vi "CheckXL_HasThisSheet.vi"(8 "error in (no error)":errorcluster, 10 "SheetName(\"\")":string, 11 "Refnum Cluster In":T1) -> (0 "error out":errorcluster, 2 "Find(False)":bool, 3 "Refnum Out":T1)   [LabVIEW 2015]
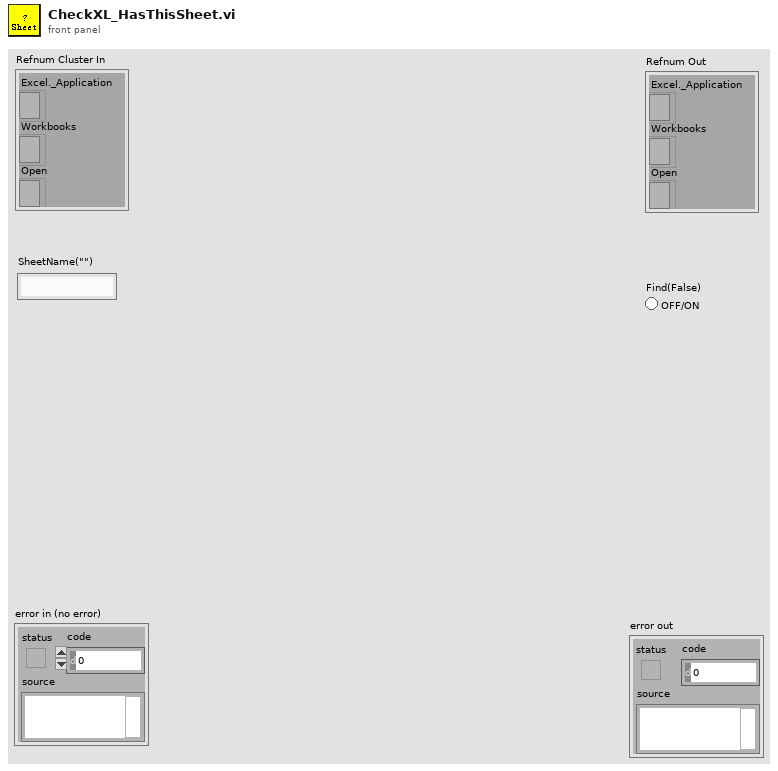
[diagram p1: front panel]
types:
  T1 = cluster{"Excel._Application":refnum<k7>, "Workbooks":refnum<k7>, "Open":refnum<k7>}
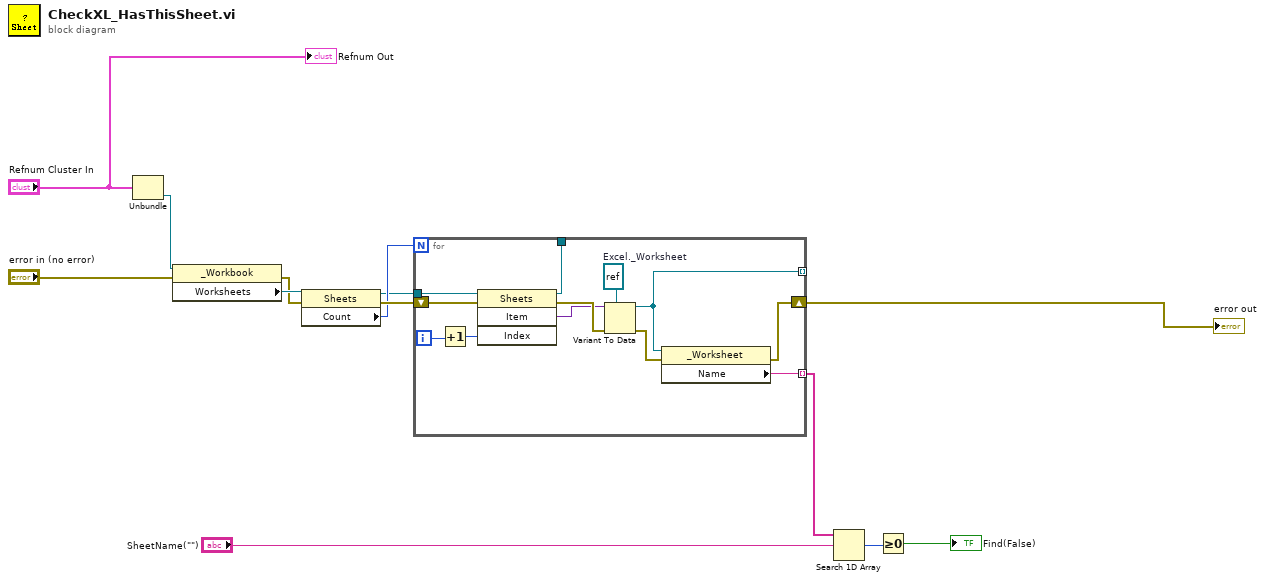
[diagram p0: block diagram]
diagram:
  n1 = Unbundle("Refnum Cluster In") -> ("Open"=w12:refnum<k7>)  [unwired: 2 out]
  n2 = property class="_Workbook"(reference=w12, error in="error in (no error)") -> (error out=w8:errorcluster, "Worksheets"=w9:refnum<k7>)  [unwired: 1 out]
  n3 = property class="Sheets"(reference=w9, error in=w8) -> (reference out=w3:refnum<k7>, error out=w7:errorcluster, "Count"=w6:i32)
  n4 = for {
    N: w6 -> [_]
    tunnel: [w25] -> _
    shift-right: [w19] -> w13
    shift-left: w7 -> [w21]
    tunnel: [w18] -> _ mode=indexing
    tunnel: [w17] -> w5 mode=indexing
    tunnel: w3 -> [w16]
    i -> [w15]
    w23 = refnum<k7> refnum  # Excel._Worksheet
    n5 = Increment(x=w15) -> (x+1=w14:i32)
    n6 = invoke class="Sheets" method="Item"(reference=w16, error in=w21, "Index"=w14) -> (reference out=w25:refnum<k7>, error out=w24:errorcluster, "Item"=w22:variant)  [unwired: 1 in, 1 out]
    n7 = Variant To Data(error in=w24, type=w23, Variant=w22) -> (data=w18:refnum<k7>, error out=w20:errorcluster)
    n8 = property class="_Worksheet"(reference=w18, error in=w20) -> (error out=w19:errorcluster, "Name"=w17:string)  [unwired: 1 out]
  }
  "error out" <- w13
  n9 = Search 1D Array(1D array=w5, element="SheetName(\"\")") -> (index of element=w2:i32)  [unwired: 1 in]
  n10 = Greater Or Equal To 0?(x=w2) -> (x >= 0?=→"Find(False)":bool)
  "Refnum Out" <- "Refnum Cluster In"
